vi "TipMap.vi"(8 "Signal":dbl format="%#_13g", 9 "Setpoint":dbl format="%#_13g", 10 "Zread":dbl format="%#_13g", 11 "Z-Position":dbl format="%#_13g") -> (1 "Tip Map":picture)   [LabVIEW 2023]
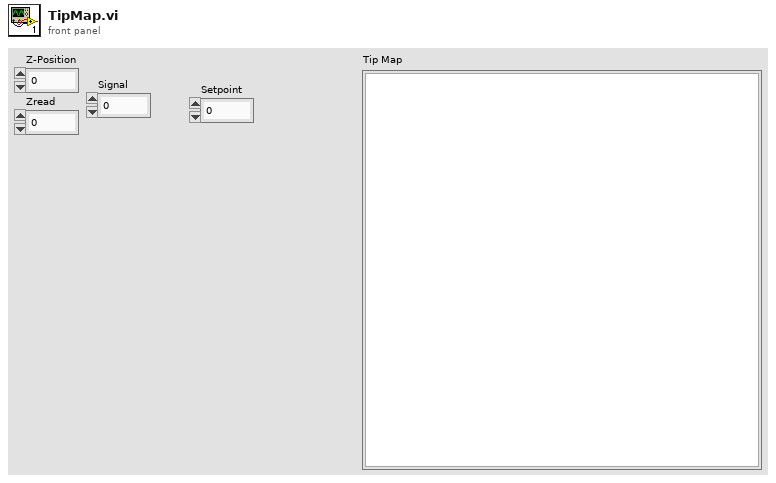
[diagram p1: front panel]
types:
  T1 = cluster{"horizontal":enum16{"left", "center", "right"}, "vertical":enum16{"top", "center", "bottom"}}
  T2 = cluster{cluster{i32, i32}, cluster{i32, i32}, cluster{i32, i32}, cluster{i32, i32}, cluster{i32, i32}, cluster{i32, i32}, cluster{i32, i32}, cluster{i32, i32}, cluster{i32, i32}, cluster{i32, i32}, cluster{i32, i32}, cluster{i32, i32}, cluster{i32, i32}, cluster{i32, i32}, cluster{i32, i32}, cluster{i32, i32}}
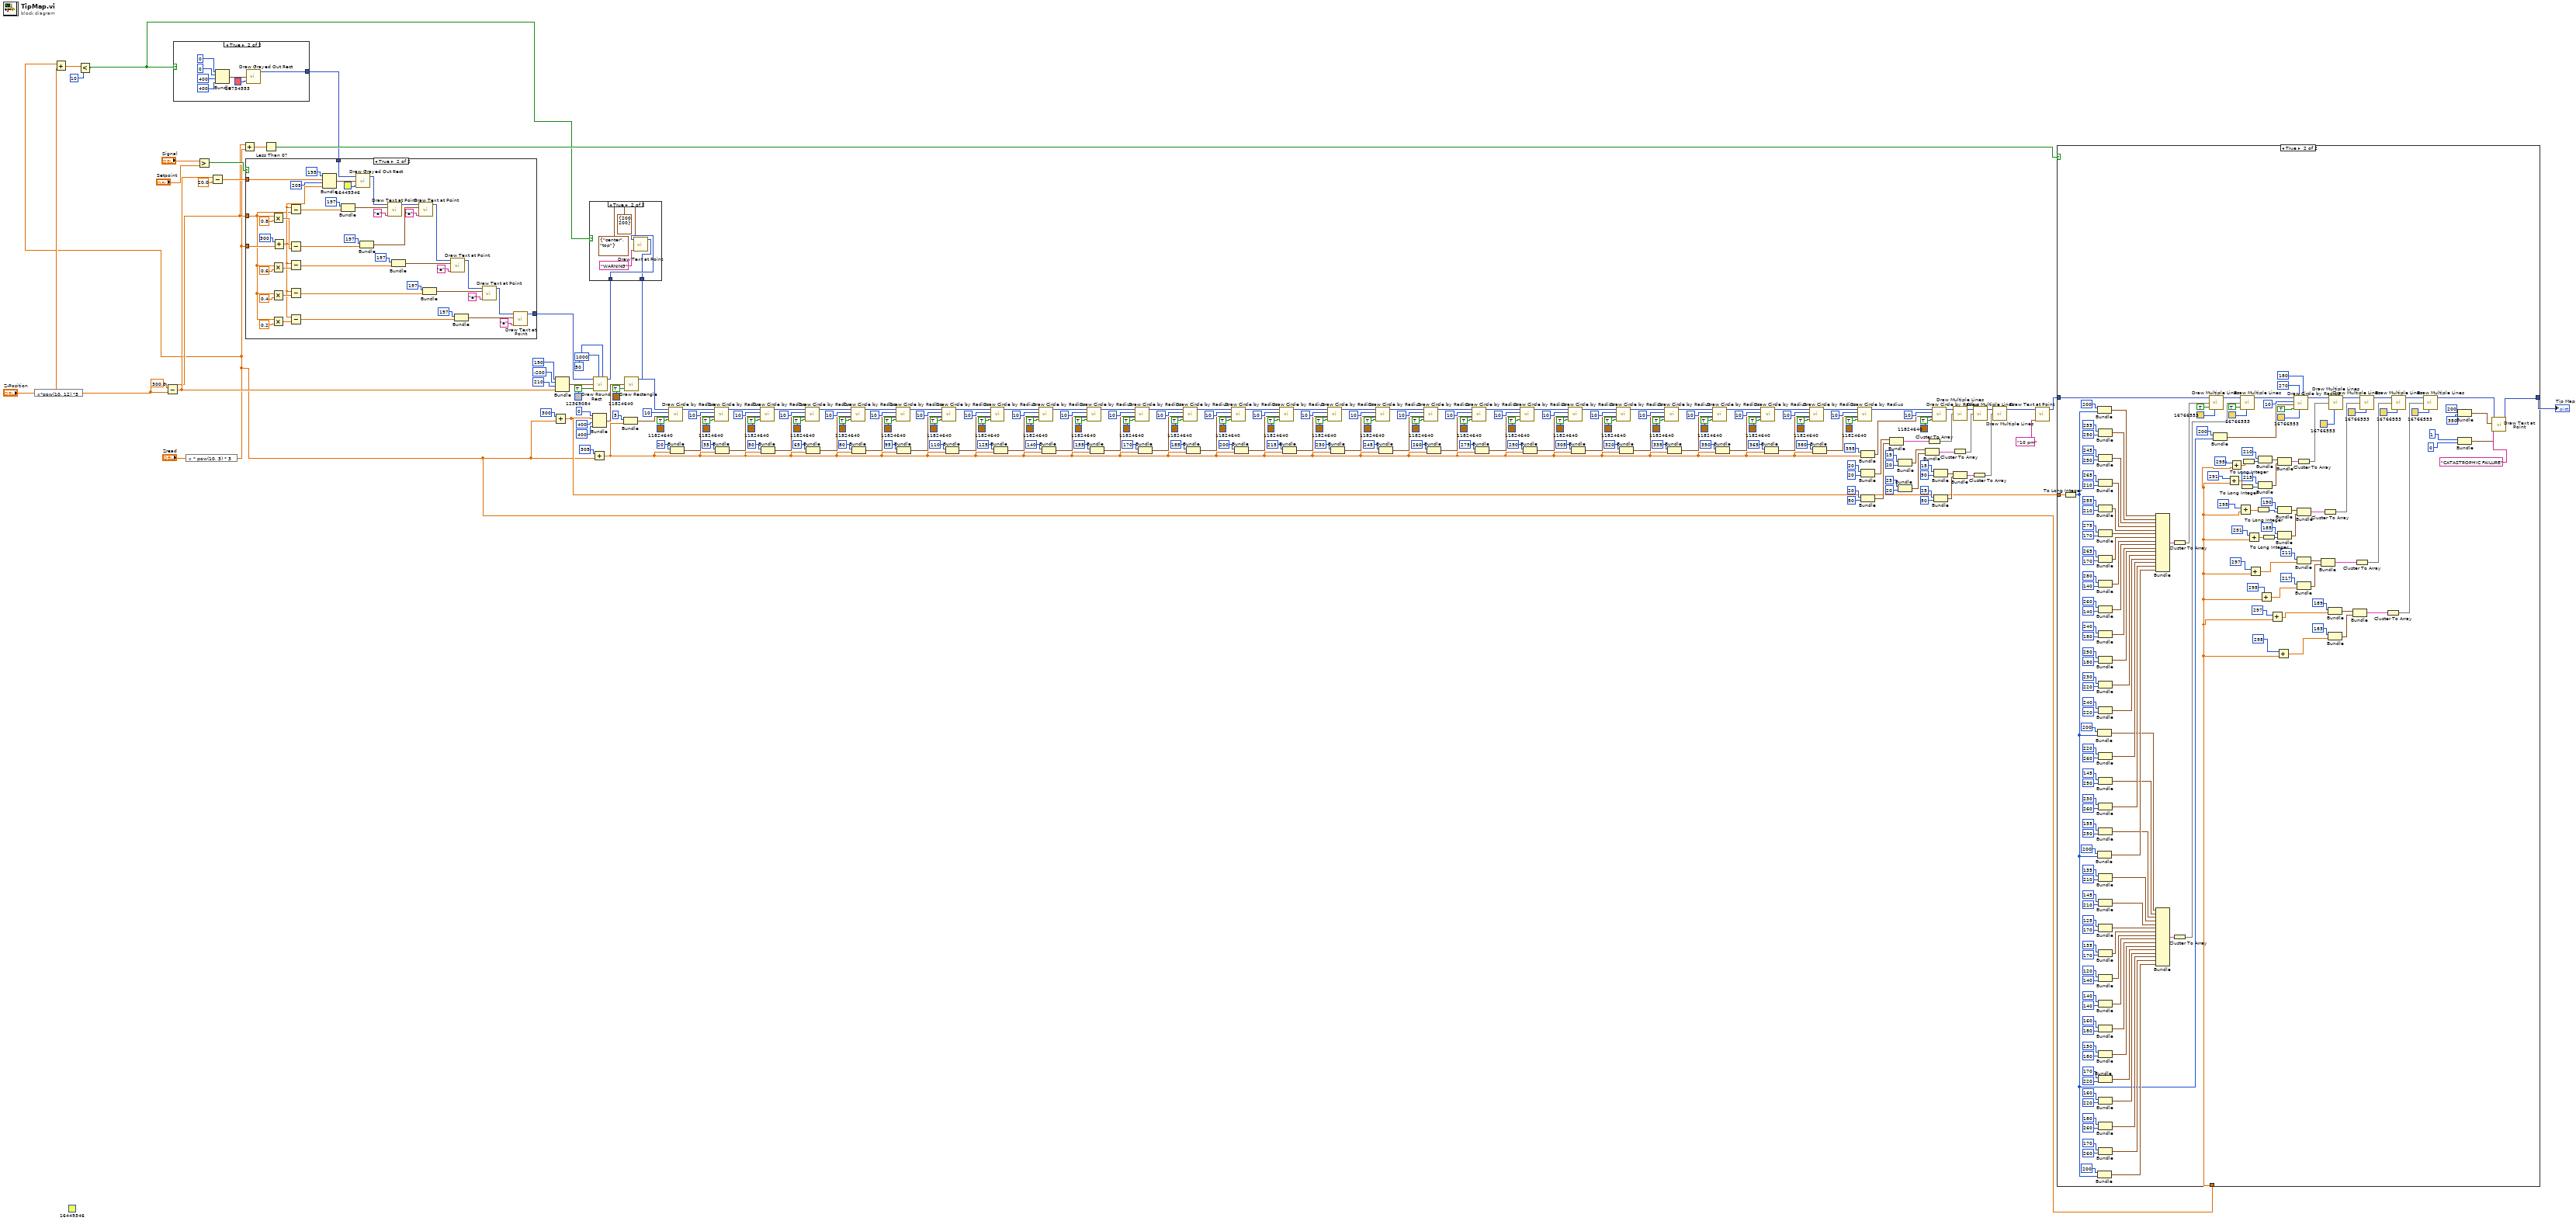
[diagram p0: block diagram]
diagram:
  (unwired) u32 16449346 ("color(black)")
  n1 = expression code="x*pow(10, 12) *3"("Z-Position") -> (w7:dbl)
  n2 = Subtract(x=300.0, y=w7) -> (x-y=w184:dbl)
  n3 = expression code="x * pow(10, 3) * 3"("Zread") -> (w6:dbl)
  n4 = Add(x=w6, y=w7) -> (x+y=w5:dbl)
  n5 = Less?(x=w5, y=10) -> (x < y?=w1:bool)
  n6 = case shown="True" w1 {
    tunnel: [_ w238] -> w8
    frame False {
    }
    frame True {
      n7 = Bundle(0, 0, 400, 400) -> (w237:cluster{i32, i32, i32, i32})  [unwired: 1 in]
      n8 = call <vilib>:"Draw Grayed Out Rect.vi"("color(black)"=u32 16734553, "rect"=w237) -> ("new picture"=w238:picture)  [unwired: 3 in]
    }
  }
  n9 = Greater?(x="Signal", y="Setpoint") -> (0:w75:bool)
  n10 = Subtract(x=w184, y=20.0) -> (x-y=w185:dbl)
  n11 = Add(x=w7, y=w6) -> (x+y=w64:dbl)
  n12 = case shown="True" w75 {
    tunnel: w185 -> [_ w278]
    tunnel: [_ w248] -> w183
    tunnel: w7 -> [_ w240]
    tunnel: w6 -> [_ w243]
    tunnel: w8 -> [_ w239]
    frame False {
    }
    frame True {
      n13 = Multiply(x=w240, y=0.8) -> (x*y=w257:dbl)
      n14 = Multiply(x=w240, y=0.6) -> (x*y=w263:dbl)
      n15 = Multiply(x=w240, y=0.4) -> (x*y=w255:dbl)
      n16 = Multiply(x=w240, y=0.2) -> (x*y=w247:dbl)
      n17 = Add(x=300, y=w243) -> (x+y=w241:dbl)
      n18 = Subtract(x=w241, y=w240) -> (x-y=w242:dbl)
      n19 = Subtract(x=w241, y=w257) -> (x-y=w269:dbl)
      n20 = Subtract(x=w241, y=w263) -> (x-y=w262:dbl)
      n21 = Subtract(x=w241, y=w255) -> (x-y=w254:dbl)
      n22 = Subtract(x=w241, y=w247) -> (x-y=w245:dbl)
      n23 = Bundle(195, w278, 205, w241) -> (w279:cluster{i32, dbl, i32, dbl})  [unwired: 1 in]
      n24 = Bundle(197, w242) -> (w276:cluster{i32, dbl})  [unwired: 1 in]
      n25 = call <vilib>:"Draw Grayed Out Rect.vi"("color(black)"=u32 16449346, "rect"=w279, "picture"=w239) -> ("new picture"=w271:picture)  [unwired: 2 in]
      n26 = Bundle(197, w269) -> (w270:cluster{i32, dbl})  [unwired: 1 in]
      n27 = call <vilib>:"Draw Text at Point.vi"("text"="e", "origin"=w276, "picture"=w271) -> ("new picture"=w272:picture)  [unwired: 7 in, 1 out]
      n28 = Bundle(197, w262) -> (w267:cluster{i32, dbl})  [unwired: 1 in]
      n29 = call <vilib>:"Draw Text at Point.vi"("text"="e", "origin"=w270, "picture"=w272) -> ("new picture"=w265:picture)  [unwired: 7 in, 1 out]
      n30 = Bundle(197, w254) -> (w260:cluster{i32, dbl})  [unwired: 1 in]
      n31 = call <vilib>:"Draw Text at Point.vi"("text"="e", "origin"=w267, "picture"=w265) -> ("new picture"=w258:picture)  [unwired: 7 in, 1 out]
      n32 = Bundle(197, w245) -> (w251:cluster{i32, dbl})  [unwired: 1 in]
      n33 = call <vilib>:"Draw Text at Point.vi"("text"="e", "origin"=w260, "picture"=w258) -> ("new picture"=w249:picture)  [unwired: 7 in, 1 out]
      n34 = call <vilib>:"Draw Text at Point.vi"("text"="e", "origin"=w251, "picture"=w249) -> ("new picture"=w248:picture)  [unwired: 7 in, 1 out]
    }
  }
  n35 = Less Than 0?(x=w64) -> (x < 0?=w216:bool)
  n36 = Add(x=300, y=w6) -> (x+y=w63:dbl)
  n37 = Bundle(190, -200, 210, w184) -> (w231:cluster{i32, i32, i32, dbl})  [unwired: 1 in]
  n38 = Bundle(0, w63, 400, 400) -> (w222:cluster{i32, dbl, i32, i32})  [unwired: 1 in]
  n39 = Add(x=i16 305 ("vertical"), y=w6) -> (x+y=w12:dbl)
  n40 = call <vilib>:"Draw Round Rect.vi"("picture"=w183, "oval width"=i16 50, "rect"=w231, "fill?(F)"=TRUE, "color(black)"=u32 12369084, "oval height"=i16 1000) -> ("new picture"=w2:picture)  [unwired: 3 in]
  n41 = case shown="True" w1 {
    tunnel: w2 -> [w283 w288]
    tunnel: [w283 w287] -> w3
    frame False {
    }
    frame True {
      n42 = call <vilib>:"Draw Text at Point.vi"("text"="WARNING", "alignment(left, top)"=T1 {"horizontal"=enum."center", "vertical"=enum."top"}, "origin"=cluster{"x":i16, "y":i16} {"x"=200, "y"=200}, "picture"=w288) -> ("new picture"=w287:picture)  [unwired: 6 in, 1 out]
    }
  }
  n43 = Bundle("horizontal"=i16 5, w12) -> (w72:cluster{"horizontal":i16, dbl})  [unwired: 1 in]
  n44 = call <vilib>:"Draw Rectangle.vi"("picture"=w3, "rect"=w222, "fill?(F)"=TRUE, "color(black)"=u32 11824640) -> ("new picture"=w51:picture)  [unwired: 5 in]
  n45 = call <vilib>:"Draw Circle by Radius.vi"("color(black)"=u32 11824640, "fill?(F)"=TRUE, "pixel center"=w72, "radius"=i16 10, "picture"=w51) -> ("new picture"=w176:picture)  [unwired: 6 in]
  n46 = Bundle("horizontal"=i16 20, w12) -> (w68:cluster{"horizontal":i16, dbl})  [unwired: 1 in]
  n47 = call <vilib>:"Draw Circle by Radius.vi"("color(black)"=u32 11824640, "fill?(F)"=TRUE, "pixel center"=w68, "radius"=i16 10, "picture"=w176) -> ("new picture"=w172:picture)  [unwired: 6 in]
  n48 = Bundle("horizontal"=i16 35, w12) -> (w66:cluster{"horizontal":i16, dbl})  [unwired: 1 in]
  n49 = call <vilib>:"Draw Circle by Radius.vi"("color(black)"=u32 11824640, "fill?(F)"=TRUE, "pixel center"=w66, "radius"=i16 10, "picture"=w172) -> ("new picture"=w168:picture)  [unwired: 6 in]
  n50 = Bundle("horizontal"=i16 50, w12) -> (w61:cluster{"horizontal":i16, dbl})  [unwired: 1 in]
  n51 = call <vilib>:"Draw Circle by Radius.vi"("color(black)"=u32 11824640, "fill?(F)"=TRUE, "pixel center"=w61, "radius"=i16 10, "picture"=w168) -> ("new picture"=w164:picture)  [unwired: 6 in]
  n52 = Bundle("horizontal"=i16 65, w12) -> (w59:cluster{"horizontal":i16, dbl})  [unwired: 1 in]
  n53 = call <vilib>:"Draw Circle by Radius.vi"("color(black)"=u32 11824640, "fill?(F)"=TRUE, "pixel center"=w59, "radius"=i16 10, "picture"=w164) -> ("new picture"=w160:picture)  [unwired: 6 in]
  n54 = Bundle("horizontal"=i16 80, w12) -> (w57:cluster{"horizontal":i16, dbl})  [unwired: 1 in]
  n55 = call <vilib>:"Draw Circle by Radius.vi"("color(black)"=u32 11824640, "fill?(F)"=TRUE, "pixel center"=w57, "radius"=i16 10, "picture"=w160) -> ("new picture"=w156:picture)  [unwired: 6 in]
  n56 = Bundle("horizontal"=i16 95, w12) -> (w55:cluster{"horizontal":i16, dbl})  [unwired: 1 in]
  n57 = call <vilib>:"Draw Circle by Radius.vi"("color(black)"=u32 11824640, "fill?(F)"=TRUE, "pixel center"=w55, "radius"=i16 10, "picture"=w156) -> ("new picture"=w152:picture)  [unwired: 6 in]
  n58 = Bundle("horizontal"=i16 110, w12) -> (w53:cluster{"horizontal":i16, dbl})  [unwired: 1 in]
  n59 = call <vilib>:"Draw Circle by Radius.vi"("color(black)"=u32 11824640, "fill?(F)"=TRUE, "pixel center"=w53, "radius"=i16 10, "picture"=w152) -> ("new picture"=w148:picture)  [unwired: 6 in]
  n60 = Bundle("horizontal"=i16 125, w12) -> (w48:cluster{"horizontal":i16, dbl})  [unwired: 1 in]
  n61 = call <vilib>:"Draw Circle by Radius.vi"("color(black)"=u32 11824640, "fill?(F)"=TRUE, "pixel center"=w48, "radius"=i16 10, "picture"=w148) -> ("new picture"=w144:picture)  [unwired: 6 in]
  n62 = Bundle("horizontal"=i16 140, w12) -> (w46:cluster{"horizontal":i16, dbl})  [unwired: 1 in]
  n63 = call <vilib>:"Draw Circle by Radius.vi"("color(black)"=u32 11824640, "fill?(F)"=TRUE, "pixel center"=w46, "radius"=i16 10, "picture"=w144) -> ("new picture"=w140:picture)  [unwired: 6 in]
  n64 = Bundle("horizontal"=i16 155, w12) -> (w44:cluster{"horizontal":i16, dbl})  [unwired: 1 in]
  n65 = call <vilib>:"Draw Circle by Radius.vi"("color(black)"=u32 11824640, "fill?(F)"=TRUE, "pixel center"=w44, "radius"=i16 10, "picture"=w140) -> ("new picture"=w136:picture)  [unwired: 6 in]
  n66 = Bundle("horizontal"=i16 170, w12) -> (w42:cluster{"horizontal":i16, dbl})  [unwired: 1 in]
  n67 = call <vilib>:"Draw Circle by Radius.vi"("color(black)"=u32 11824640, "fill?(F)"=TRUE, "pixel center"=w42, "radius"=i16 10, "picture"=w136) -> ("new picture"=w132:picture)  [unwired: 6 in]
  n68 = Bundle("horizontal"=i16 185, w12) -> (w40:cluster{"horizontal":i16, dbl})  [unwired: 1 in]
  n69 = call <vilib>:"Draw Circle by Radius.vi"("color(black)"=u32 11824640, "fill?(F)"=TRUE, "pixel center"=w40, "radius"=i16 10, "picture"=w132) -> ("new picture"=w128:picture)  [unwired: 6 in]
  n70 = Bundle("horizontal"=i16 200, w12) -> (w38:cluster{"horizontal":i16, dbl})  [unwired: 1 in]
  n71 = call <vilib>:"Draw Circle by Radius.vi"("color(black)"=u32 11824640, "fill?(F)"=TRUE, "pixel center"=w38, "radius"=i16 10, "picture"=w128) -> ("new picture"=w124:picture)  [unwired: 6 in]
  n72 = Bundle("horizontal"=i16 215, w12) -> (w36:cluster{"horizontal":i16, dbl})  [unwired: 1 in]
  n73 = call <vilib>:"Draw Circle by Radius.vi"("color(black)"=u32 11824640, "fill?(F)"=TRUE, "pixel center"=w36, "radius"=i16 10, "picture"=w124) -> ("new picture"=w120:picture)  [unwired: 6 in]
  n74 = Bundle("horizontal"=i16 230, w12) -> (w34:cluster{"horizontal":i16, dbl})  [unwired: 1 in]
  n75 = call <vilib>:"Draw Circle by Radius.vi"("color(black)"=u32 11824640, "fill?(F)"=TRUE, "pixel center"=w34, "radius"=i16 10, "picture"=w120) -> ("new picture"=w116:picture)  [unwired: 6 in]
  n76 = Bundle("horizontal"=i16 245, w12) -> (w32:cluster{"horizontal":i16, dbl})  [unwired: 1 in]
  n77 = call <vilib>:"Draw Circle by Radius.vi"("color(black)"=u32 11824640, "fill?(F)"=TRUE, "pixel center"=w32, "radius"=i16 10, "picture"=w116) -> ("new picture"=w112:picture)  [unwired: 6 in]
  n78 = Bundle("horizontal"=i16 260, w12) -> (w30:cluster{"horizontal":i16, dbl})  [unwired: 1 in]
  n79 = call <vilib>:"Draw Circle by Radius.vi"("color(black)"=u32 11824640, "fill?(F)"=TRUE, "pixel center"=w30, "radius"=i16 10, "picture"=w112) -> ("new picture"=w109:picture)  [unwired: 6 in]
  n80 = Bundle("horizontal"=i16 275, w12) -> (w28:cluster{"horizontal":i16, dbl})  [unwired: 1 in]
  n81 = call <vilib>:"Draw Circle by Radius.vi"("color(black)"=u32 11824640, "fill?(F)"=TRUE, "pixel center"=w28, "radius"=i16 10, "picture"=w109) -> ("new picture"=w105:picture)  [unwired: 6 in]
  n82 = Bundle("horizontal"=i16 290, w12) -> (w26:cluster{"horizontal":i16, dbl})  [unwired: 1 in]
  n83 = call <vilib>:"Draw Circle by Radius.vi"("color(black)"=u32 11824640, "fill?(F)"=TRUE, "pixel center"=w26, "radius"=i16 10, "picture"=w105) -> ("new picture"=w101:picture)  [unwired: 6 in]
  n84 = Bundle("horizontal"=i16 305, w12) -> (w24:cluster{"horizontal":i16, dbl})  [unwired: 1 in]
  n85 = call <vilib>:"Draw Circle by Radius.vi"("color(black)"=u32 11824640, "fill?(F)"=TRUE, "pixel center"=w24, "radius"=i16 10, "picture"=w101) -> ("new picture"=w97:picture)  [unwired: 6 in]
  n86 = Bundle("horizontal"=i16 320, w12) -> (w22:cluster{"horizontal":i16, dbl})  [unwired: 1 in]
  n87 = call <vilib>:"Draw Circle by Radius.vi"("color(black)"=u32 11824640, "fill?(F)"=TRUE, "pixel center"=w22, "radius"=i16 10, "picture"=w97) -> ("new picture"=w93:picture)  [unwired: 6 in]
  n88 = Bundle("horizontal"=i16 335, w12) -> (w20:cluster{"horizontal":i16, dbl})  [unwired: 1 in]
  n89 = call <vilib>:"Draw Circle by Radius.vi"("color(black)"=u32 11824640, "fill?(F)"=TRUE, "pixel center"=w20, "radius"=i16 10, "picture"=w93) -> ("new picture"=w89:picture)  [unwired: 6 in]
  n90 = Bundle("horizontal"=i16 350, w12) -> (w18:cluster{"horizontal":i16, dbl})  [unwired: 1 in]
  n91 = call <vilib>:"Draw Circle by Radius.vi"("color(black)"=u32 11824640, "fill?(F)"=TRUE, "pixel center"=w18, "radius"=i16 10, "picture"=w89) -> ("new picture"=w85:picture)  [unwired: 6 in]
  n92 = Bundle("horizontal"=i16 365, w12) -> (w16:cluster{"horizontal":i16, dbl})  [unwired: 1 in]
  n93 = call <vilib>:"Draw Circle by Radius.vi"("color(black)"=u32 11824640, "fill?(F)"=TRUE, "pixel center"=w16, "radius"=i16 10, "picture"=w85) -> ("new picture"=w81:picture)  [unwired: 6 in]
  n94 = Bundle("horizontal"=i16 380, w12) -> (w14:cluster{"horizontal":i16, dbl})  [unwired: 1 in]
  n95 = call <vilib>:"Draw Circle by Radius.vi"("color(black)"=u32 11824640, "fill?(F)"=TRUE, "pixel center"=w14, "radius"=i16 10, "picture"=w81) -> ("new picture"=w52:picture)  [unwired: 6 in]
  n96 = Bundle("horizontal"=i16 395, w12) -> (w11:cluster{"horizontal":i16, dbl})  [unwired: 1 in]
  n97 = Bundle(20, 20) -> (w211:cluster{i32, i32})  [unwired: 1 in]
  n98 = Bundle(20, 50) -> (w210:cluster{i32, i32})  [unwired: 1 in]
  n99 = Bundle(w211, w210) -> (w209:cluster{cluster{i32, i32}, cluster{i32, i32}})  [unwired: 1 in]
  n100 = Bundle(15, 20) -> (w203:cluster{i32, i32})  [unwired: 1 in]
  n101 = Bundle(25, 20) -> (w202:cluster{i32, i32})  [unwired: 1 in]
  n102 = Bundle(w203, w202) -> (w201:cluster{cluster{i32, i32}, cluster{i32, i32}})  [unwired: 1 in]
  n103 = Cluster To Array(cluster=w209) -> (array=w208:cluster{i32, i32}[])
  n104 = call <vilib>:"Draw Circle by Radius.vi"("color(black)"=u32 11824640, "fill?(F)"=TRUE, "pixel center"=w11, "radius"=i16 10, "picture"=w52) -> ("new picture"=w50:picture)  [unwired: 6 in]
  n105 = Bundle(15, 50) -> (w194:cluster{i32, i32})  [unwired: 1 in]
  n106 = Bundle(25, 50) -> (w193:cluster{i32, i32})  [unwired: 1 in]
  n107 = Cluster To Array(cluster=w201) -> (array=w200:cluster{i32, i32}[])
  n108 = call <vilib>:"Draw Multiple Lines.vi"("picture"=w50, "line endpoints"=w208) -> ("new picture"=w199:picture)  [unwired: 7 in]
  n109 = Bundle(w194, w193) -> (w192:cluster{cluster{i32, i32}, cluster{i32, i32}})  [unwired: 1 in]
  n110 = Cluster To Array(cluster=w192) -> (array=w191:cluster{i32, i32}[])
  n111 = call <vilib>:"Draw Multiple Lines.vi"("picture"=w199, "line endpoints"=w200) -> ("new picture"=w190:picture)  [unwired: 7 in]
  n112 = call <vilib>:"Draw Multiple Lines.vi"("picture"=w190, "line endpoints"=w191) -> ("new picture"=w189:picture)  [unwired: 7 in]
  n113 = call <vilib>:"Draw Text at Point.vi"("text"="10 pm", "picture"=w189) -> ("new picture"=w187:picture)  [unwired: 8 in, 1 out]
  n114 = case shown="True" w216 {
    tunnel: [w289 w297] -> w217
    tunnel: w187 -> [w289 w325]
    tunnel: w63 -> [_ w324]
    tunnel: w6 -> [_ w301]
    frame False {
    }
    frame True {
      n115 = To Long Integer(number=w324) -> (32bit integer=w319:i32)
      n116 = Bundle(200, w319) -> (w458:cluster{i32, i32})  [unwired: 1 in]
      n117 = Bundle(200, w319) -> (w408:cluster{i32, i32})  [unwired: 1 in]
      n118 = Bundle(200, w319) -> (w415:cluster{i32, i32})  [unwired: 1 in]
      n119 = Bundle(200, w319) -> (w365:cluster{i32, i32})  [unwired: 1 in]
      n120 = Bundle(255, 250) -> (w457:cluster{i32, i32})  [unwired: 1 in]
      n121 = Bundle(245, 250) -> (w456:cluster{i32, i32})  [unwired: 1 in]
      n122 = Bundle(265, 210) -> (w450:cluster{i32, i32})  [unwired: 1 in]
      n123 = Bundle(255, 210) -> (w447:cluster{i32, i32})  [unwired: 1 in]
      n124 = Bundle(275, 170) -> (w444:cluster{i32, i32})  [unwired: 1 in]
      n125 = Bundle(265, 170) -> (w441:cluster{i32, i32})  [unwired: 1 in]
      n126 = Bundle(280, 140) -> (w438:cluster{i32, i32})  [unwired: 1 in]
      n127 = Bundle(260, 140) -> (w435:cluster{i32, i32})  [unwired: 1 in]
      n128 = Bundle(240, 180) -> (w432:cluster{i32, i32})  [unwired: 1 in]
      n129 = Bundle(250, 180) -> (w429:cluster{i32, i32})  [unwired: 1 in]
      n130 = Bundle(230, 220) -> (w426:cluster{i32, i32})  [unwired: 1 in]
      n131 = Bundle(240, 220) -> (w423:cluster{i32, i32})  [unwired: 1 in]
      n132 = Bundle(220, 260) -> (w420:cluster{i32, i32})  [unwired: 1 in]
      n133 = Bundle(145, 250) -> (w407:cluster{i32, i32})  [unwired: 1 in]
      n134 = Bundle(230, 260) -> (w417:cluster{i32, i32})  [unwired: 1 in]
      n135 = Bundle(155, 250) -> (w406:cluster{i32, i32})  [unwired: 1 in]
      n136 = Bundle(135, 210) -> (w400:cluster{i32, i32})  [unwired: 1 in]
      n137 = Bundle(145, 210) -> (w397:cluster{i32, i32})  [unwired: 1 in]
      n138 = Bundle(125, 170) -> (w394:cluster{i32, i32})  [unwired: 1 in]
      n139 = Bundle(135, 170) -> (w391:cluster{i32, i32})  [unwired: 1 in]
      n140 = Bundle(120, 140) -> (w388:cluster{i32, i32})  [unwired: 1 in]
      n141 = Bundle(140, 140) -> (w385:cluster{i32, i32})  [unwired: 1 in]
      n142 = Bundle(160, 180) -> (w382:cluster{i32, i32})  [unwired: 1 in]
      n143 = Bundle(150, 180) -> (w379:cluster{i32, i32})  [unwired: 1 in]
      n144 = Bundle(170, 220) -> (w376:cluster{i32, i32})  [unwired: 1 in]
      n145 = Bundle(160, 220) -> (w373:cluster{i32, i32})  [unwired: 1 in]
      n146 = Bundle(180, 260) -> (w370:cluster{i32, i32})  [unwired: 1 in]
      n147 = Bundle(170, 260) -> (w367:cluster{i32, i32})  [unwired: 1 in]
      n148 = Bundle(w458, w457, w456, w450, w447, w444, w441, w438, w435, w432, w429, w426, w423, w420, w417, w415) -> (w455:T2)  [unwired: 1 in]
      n149 = Bundle(w408, w407, w406, w400, w397, w394, w391, w388, w385, w382, w379, w376, w373, w370, w367, w365) -> (w405:T2)  [unwired: 1 in]
      n150 = Cluster To Array(cluster=w455) -> (array=w454:cluster{i32, i32}[])
      n151 = Cluster To Array(cluster=w405) -> (array=w404:cluster{i32, i32}[])
      n152 = call <vilib>:"Draw Multiple Lines.vi"("picture"=w325, "line endpoints"=w454, "fill?(F)"=TRUE, "color(black)"=u32 16766553) -> ("new picture"=w364:picture)  [unwired: 5 in]
      n153 = Bundle("horizontal"=i16 200, w319) -> (w322:cluster{"horizontal":i16, i32})  [unwired: 1 in]
      n154 = Add(x=291, y=w301) -> (x+y=w318:dbl)
      n155 = Add(x=295, y=w301) -> (x+y=w317:dbl)
      n156 = Add(x=295, y=w301) -> (x+y=w314:dbl)
      n157 = To Long Integer(number=w318) -> (32bit integer=w316:i32)
      n158 = call <vilib>:"Draw Multiple Lines.vi"("picture"=w364, "line endpoints"=w404, "fill?(F)"=TRUE, "color(black)"=u32 16766553) -> ("new picture"=w362:picture)  [unwired: 5 in]
      n159 = To Long Integer(number=w317) -> (32bit integer=w315:i32)
      n160 = Add(x=291, y=w301) -> (x+y=w310:dbl)
      n161 = Add(x=297, y=w301) -> (x+y=w308:dbl)
      n162 = To Long Integer(number=w314) -> (32bit integer=w312:i32)
      n163 = Bundle(210, w315) -> (w354:cluster{i32, i32})  [unwired: 1 in]
      n164 = Bundle(215, w316) -> (w353:cluster{i32, i32})  [unwired: 1 in]
      n165 = Add(x=295, y=w301) -> (x+y=w305:dbl)
      n166 = To Long Integer(number=w310) -> (32bit integer=w309:i32)
      n167 = Add(x=297, y=w301) -> (x+y=w303:dbl)
      n168 = Add(x=295, y=w301) -> (x+y=w300:dbl)
      n169 = Bundle(190, w312) -> (w347:cluster{i32, i32})  [unwired: 1 in]
      n170 = Bundle(185, w309) -> (w346:cluster{i32, i32})  [unwired: 1 in]
      n171 = Bundle(w354, w353) -> (w352:cluster{cluster{i32, i32}, cluster{i32, i32}})  [unwired: 1 in]
      n172 = call <vilib>:"Draw Circle by Radius.vi"("arc size(360)"=i16 180, "color(black)"=u32 16766553, "start angle(0)"=i16 270, "fill?(F)"=TRUE, "pixel center"=w322, "radius"=i16 10, "picture"=w362) -> ("new picture"=w350:picture)  [unwired: 4 in]
      n173 = Cluster To Array(cluster=w352) -> (array=w351:cluster{i32, i32}[])
      n174 = Bundle(211, w308) -> (w340:cluster{i32, dbl})  [unwired: 1 in]
      n175 = Bundle(217, w305) -> (w339:cluster{i32, dbl})  [unwired: 1 in]
      n176 = Bundle(w347, w346) -> (w345:cluster{cluster{i32, i32}, cluster{i32, i32}})  [unwired: 1 in]
      n177 = Bundle(w340, w339) -> (w338:cluster{cluster{i32, dbl}, cluster{i32, dbl}})  [unwired: 1 in]
      n178 = Cluster To Array(cluster=w345) -> (array=w344:cluster{i32, i32}[])
      n179 = Bundle(189, w303) -> (w333:cluster{i32, dbl})  [unwired: 1 in]
      n180 = Bundle(183, w300) -> (w332:cluster{i32, dbl})  [unwired: 1 in]
      n181 = call <vilib>:"Draw Multiple Lines.vi"("picture"=w350, "line endpoints"=w351, "color(black)"=u32 16766553) -> ("new picture"=w343:picture)  [unwired: 6 in]
      n182 = Bundle(w333, w332) -> (w331:cluster{cluster{i32, dbl}, cluster{i32, dbl}})  [unwired: 1 in]
      n183 = Cluster To Array(cluster=w338) -> (array=w337:cluster{i32, dbl}[])
      n184 = call <vilib>:"Draw Multiple Lines.vi"("picture"=w343, "line endpoints"=w344, "color(black)"=u32 16766553) -> ("new picture"=w336:picture)  [unwired: 6 in]
      n185 = Cluster To Array(cluster=w331) -> (array=w330:cluster{i32, dbl}[])
      n186 = call <vilib>:"Draw Multiple Lines.vi"("picture"=w336, "line endpoints"=w337, "color(black)"=u32 16766553) -> ("new picture"=w329:picture)  [unwired: 6 in]
      n187 = call <vilib>:"Draw Multiple Lines.vi"("picture"=w329, "line endpoints"=w330, "color(black)"=u32 16766553) -> ("new picture"=w298:picture)  [unwired: 6 in]
      n188 = Bundle(200, 350) -> (w295:cluster{i32, i32})  [unwired: 1 in]
      n189 = Bundle(1, 0) -> (w292:cluster{i32, i32})  [unwired: 1 in]
      n190 = call <vilib>:"Draw Text at Point.vi"("text"="CATASTROPHIC FAILURE", "alignment(left, top)"=w292, "origin"=w295, "picture"=w298) -> ("new picture"=w297:picture)  [unwired: 6 in, 1 out]
    }
  }
  "Tip Map" <- w217
